vi "Queue Status Conditional.vi"(8 "error in (no error)":errorcluster, 11 "Queue in":refnum<queue>) -> (0 "error out":errorcluster, 3 "Queue out":refnum<queue>)   [LabVIEW 2020]
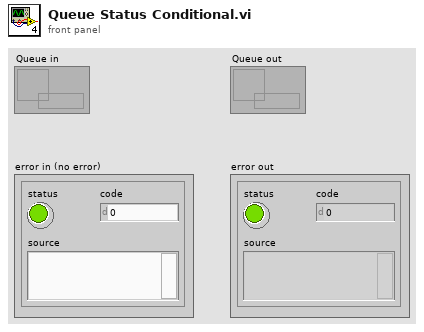
[diagram p1: front panel]
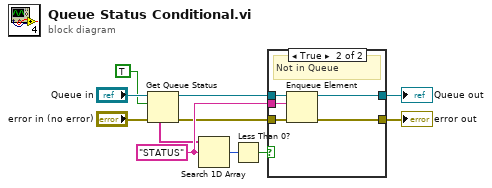
[diagram p0: block diagram]
diagram:
  w9 = "STATUS" ("element")
  n1 = Get Queue Status(queue="Queue in", return elements? (F)=TRUE, error in (no error)="error in (no error)") -> (queue out=w3:refnum<queue>, error out=w2:errorcluster, elements=w4:string[])  [unwired: 5 out]
  n2 = Search 1D Array(1D array=w4, element=w9) -> (index of element=w8:i32)  [unwired: 1 in]
  n3 = Less Than 0?(x=w8) -> (x < 0?=w7:bool)
  n4 = case shown="True" w7 {
    tunnel: w3 -> [w13 w18]
    tunnel: w2 -> [w12 w17]
    tunnel: w9 -> [_ w16]
    tunnel: [w13 w15] -> w11
    tunnel: [w12 w14] -> w10
    frame False {
      # "Already in Queue"
    }
    frame True {
      # "Not in Queue"
      n5 = Enqueue Element(queue=w18, element=w16, error in (no error)=w17) -> (queue out=w15:refnum<queue>, error out=w14:errorcluster)  [unwired: 1 in, 1 out]
    }
  }
  "Queue out" <- w11
  "error out" <- w10
